vi "Unit Test - Copy Specified State.vi"() -> (3 "Array":T1(array[cluster])=[{"state"="Idle", "error out"={"status"=FALSE, "code"=0, "source"=""}, "Execution:State"=enum."Idle"}, {"state"="CSM Documentation", "error out"={"status"=FALSE, "code"=0, "source"=""}, "Execution:State"=enum."Idle"}, {"state"="VI Reference", "error out"={"status"=FALSE, "code"=0, "source"=""}, "Execution:State"=enum."Idle"}, {"state"="Error Handler", "error out"={"status"=FALSE, "code"=0, "source"=""}, "Execution:State"=enum."Bad"}, {"state"="Critical Error", "error out"={"status"=FALSE, "code"=0, "source"=""}, "Execution:State"=enum."Idle"}, {"state"="Target Timeout Error", "error out"={"status"=FALSE, "code"=0, "source"=""}, "Execution:State"=enum."Idle"}, {"state"="Target Error", "error out"={"status"=FALSE, "code"=0, "source"=""}, "Execution:State"=enum."Idle"}, {"state"="Async Response", "error out"={"status"=FALSE, "code"=0, "source"=""}, "Execution:State"=enum."Idle"}, {"state"="Response", "error out"={"status"=FALSE, "code"=0, "source"=""}, "Execution:State"=enum."Idle"}, {"state"="Async Message Posted", "error out"={"status"=FALSE, "code"=0, "source"=""}, "Execution:State"=enum."Idle"}, {"state"="Initialize Core Data", "error out"={"status"=FALSE, "code"=0, "source"=""}, "Execution:State"=enum."Idle"}, {"state"="Exit", "error out"={"status"=FALSE, "code"=0, "source"=""}, "Execution:State"=enum."Idle"}, {"state"="Data: Initialize", "error out"={"status"=FALSE, "code"=0, "source"=""}, "Execution:State"=enum."Idle"}, {"state"="Data: Update Indicators", "error out"={"status"=FALSE, "code"=0, "source"=""}, "Execution:State"=enum."Idle"}, {"state"="Data: Cleanup", "error out"={"status"=FALSE, "code"=0, "source"=""}, "Execution:State"=enum."Idle"}, {"state"="Macro: Initialize", "error out"={"status"=FALSE, "code"=0, "source"=""}, "Execution:State"=enum."Idle"}, {"state"="Macro: Exit", "error out"={"status"=FALSE, "code"=0, "source"=""}, "Execution:State"=enum."Idle"}, {"state"="API: API1", "error out"={"status"=FALSE, "code"=0, "source"=""}, "Execution:State"=enum."Idle"}, {"state"="API: API2", "error out"={"status"=FALSE, "code"=0, "source"=""}, "Execution:State"=enum."Idle"}, {"state"="Action: action1", "error out"={"status"=FALSE, "code"=0, "source"=""}, "Execution:State"=enum."Idle"}, {"state"="Action: action2", "error out"={"status"=FALSE, "code"=0, "source"=""}, "Execution:State"=enum."Idle"}])   [LabVIEW 2017, in "testcase-csmhelper.lvclass"]
uses:
  testcase-csmhelper.lvclass
  src/user.lib/_NEVSTOP/Communicable State Machine(CSM)/_csmHelper/CSM-Helper.lvclass/CSM-Helper.ctl
  src/user.lib/_NEVSTOP/Communicable State Machine(CSM)/_csmHelper/Properties/Read VI Ref.vi
  src/user.lib/_NEVSTOP/Communicable State Machine(CSM)/_csmHelper/API/Create From VI Reference.vi
  src/user.lib/_NEVSTOP/Communicable State Machine(CSM)/_csmHelper/API/Start Undo.vi
  src/user.lib/_NEVSTOP/Communicable State Machine(CSM)/_csmHelper/API/Copy State.vi
  src/user.lib/_NEVSTOP/Communicable State Machine(CSM)/_csmHelper/API/Stop Undo.vi
  src/user.lib/_NEVSTOP/Communicable State Machine(CSM)/_csmHelper/API/Undo.vi
  src/user.lib/_NEVSTOP/Communicable State Machine(CSM)/_csmHelper/API/Destroy.vi
  src/user.lib/_NEVSTOP/Communicable State Machine(CSM)/_csmHelper/CSM-Helper.lvclass
  src/user.lib/_NEVSTOP/Communicable State Machine(CSM)/_csmHelper/API/Open Block Diagram.vi
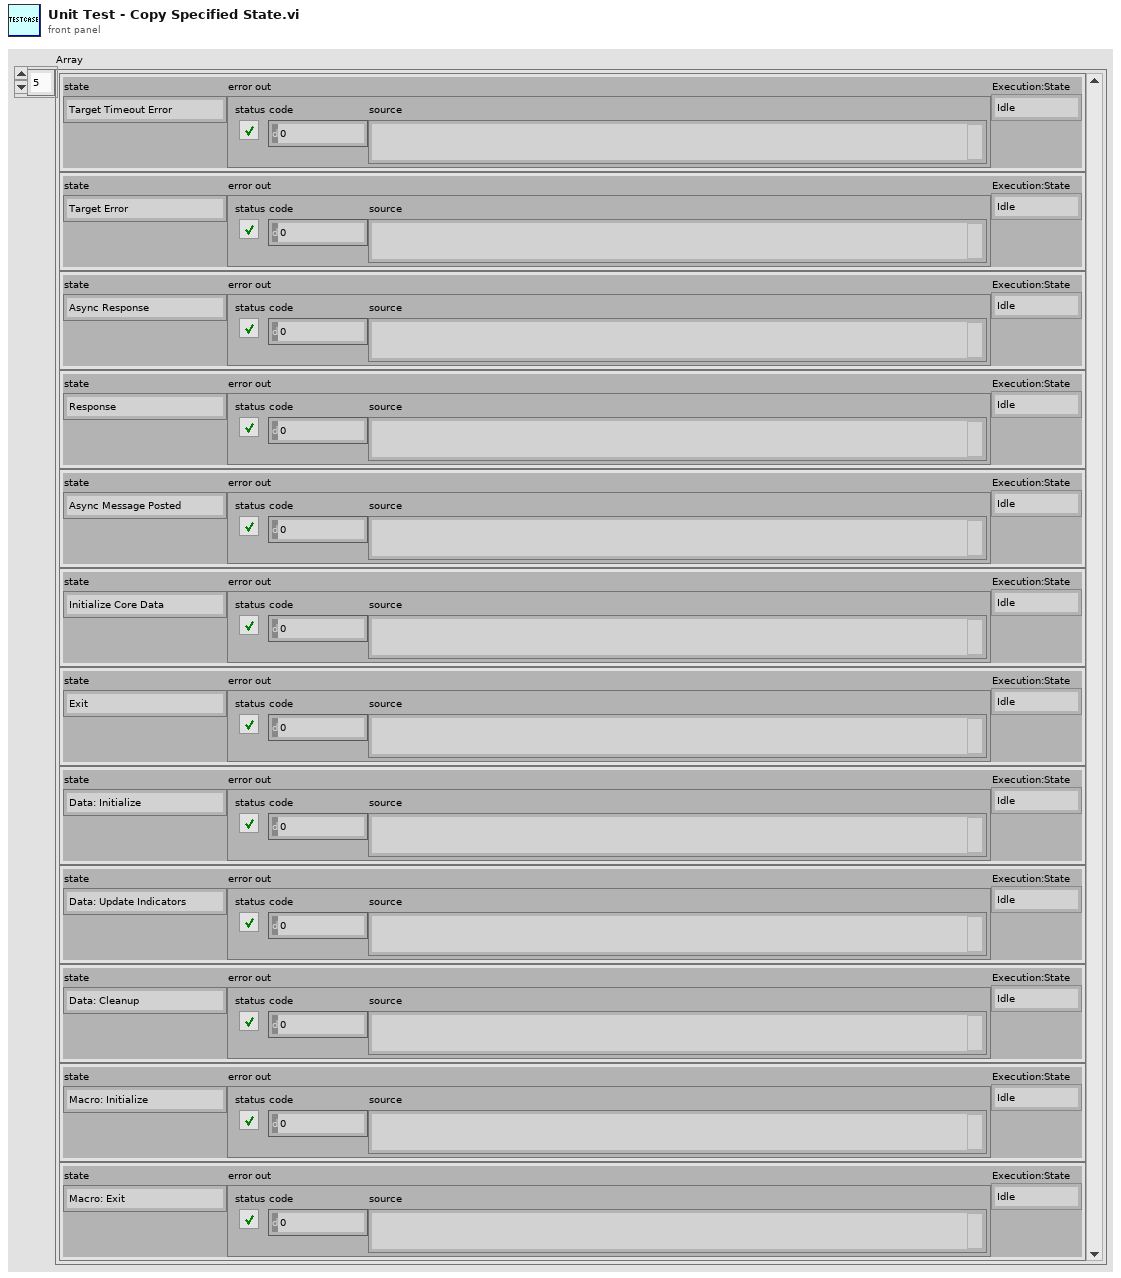
[diagram p1: front panel]
types:
  T1 = cluster{"state":string, "error out":errorcluster, "Execution:State":enum32{"Bad", "Idle", "Run top level", "Running"}}[]
  T2 = enum32{"Bad", "Idle", "Run top level", "Running"}
  T3 = cluster{string, "error out":errorcluster, "Exec.State":enum32{"Bad", "Idle", "Run top level", "Running"}}
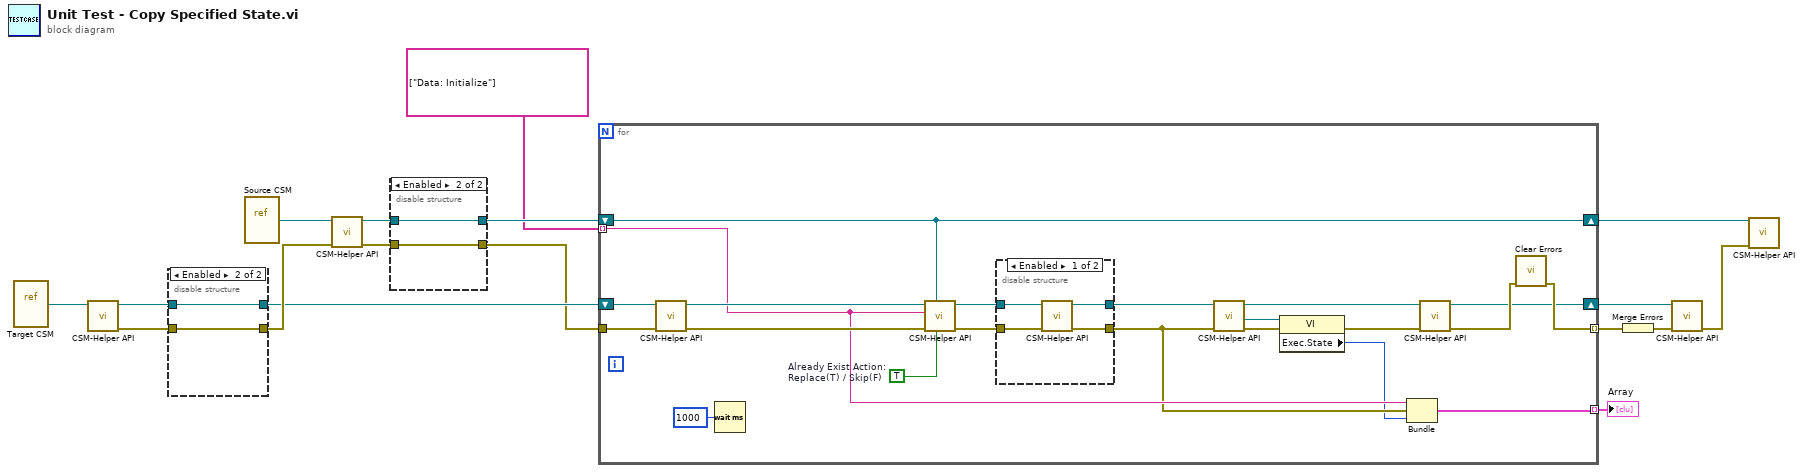
[diagram p0: block diagram]
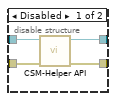
[diagram p2: hidden frame]
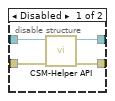
[diagram p3: hidden frame]
diagram:
  n1 = vi-ref "Target CSM.vi"() -> (w1:refnum<vi>)
  n2 = call-poly "CSM-Helper API.vi"("VI"=w1) -> ("error out"=w15:errorcluster, "CSM-Helper.lvclass"=w14:refnum<class "CSM-Helper.lvclass">)  [unwired: 9 in]
  n3 = disable-structure shown="Enabled" {
    disable-tunnel: w15 -> [w21 w22]
    disable-tunnel: w14 -> [w20 w23]
    disable-tunnel: [w19 w22] -> w11
    disable-tunnel: [w18 w23] -> w10
    frame Disabled {
      n4 = call-poly "CSM-Helper API.vi"("error in (no error)"=w21, "CSM-Helper in"=w20) -> ("error out"=w19:errorcluster, "CSM-Helper out"=w18:refnum<class "CSM-Helper.lvclass">)  [unwired: 8 in]
    }
    frame Enabled {
    }
  }
  n5 = vi-ref "Source CSM.vi"() -> (w2:refnum<vi>)
  n6 = call-poly "CSM-Helper API.vi"("error in (no error)"=w11, "VI"=w2) -> ("error out"=w12:errorcluster, "CSM-Helper.lvclass"=w13:refnum<class "CSM-Helper.lvclass">)  [unwired: 8 in]
  n7 = disable-structure shown="Enabled" {
    disable-tunnel: w13 -> [w27 w29]
    disable-tunnel: w12 -> [w26 w28]
    disable-tunnel: [w25 w29] -> w5
    disable-tunnel: [w24 w28] -> w4
    frame Disabled {
      n8 = call-poly "CSM-Helper API.vi"("error in (no error)"=w26, "CSM-Helper in"=w27) -> ("error out"=w24:errorcluster, "CSM-Helper out"=w25:refnum<class "CSM-Helper.lvclass">)  [unwired: 8 in]
    }
    frame Enabled {
    }
  }
  n9 = for {
    shift-right: [w38] -> w17
    shift-left: w10 -> [w49]
    shift-right: [w44] -> w8
    shift-left: w5 -> [w44]
    tunnel: string[] ["Data: Initialize"] ("Value") -> [w42] mode=indexing
    tunnel: w4 -> [w48]
    tunnel: [w43] -> w16 mode=indexing
    tunnel: [w41] -> w6 mode=indexing
    w30 = TRUE  # Already Exist Action: Replace(T) / Skip(F)
    n10 = call-poly "CSM-Helper API.vi"("error in (no error)"=w48, "CSM-Helper in"=w49) -> ("error out"=w47:errorcluster, "CSM-Helper out"=w46:refnum<class "CSM-Helper.lvclass">)  [unwired: 8 in]
    n11 = Wait (ms)(milliseconds to wait=u32 1000) -> ()  [unwired: 1 out]
    n12 = call-poly "CSM-Helper API.vi"("Already Exist Action:\nReplace(T) / Skip(F)"=w30, "SourceCSM"=w44, "error in (no error)"=w47, "Case"=w42, "CSM-Helper.lvclass"=w46) -> ("error out"=w45:errorcluster, "CSM-Helper out 2"=w50:refnum<class "CSM-Helper.lvclass">)  [unwired: 5 in]
    n13 = disable-structure shown="Enabled" {
      disable-tunnel: [w54 w56] -> w36
      disable-tunnel: w45 -> [w53 w55]
      disable-tunnel: [w52 w55] -> w37
      disable-tunnel: w50 -> [w51 w56]
      frame Enabled {
        n14 = call-poly "CSM-Helper API.vi"("error in (no error)"=w53, "CSM-Helper in"=w51) -> ("error out"=w52:errorcluster, "CSM-Helper out"=w54:refnum<class "CSM-Helper.lvclass">)  [unwired: 8 in]
      }
      frame Disabled {
      }
    }
    n15 = call-poly "CSM-Helper API.vi"("error in (no error)"=w37, "CSM-Helper in"=w36) -> ("error out"=w34:errorcluster, "VI"=w32:refnum<vi>, "CSM-Helper out"=w35:refnum<class "CSM-Helper.lvclass">)  [unwired: 7 in]
    n16 = property class="VI"(reference=w32, error in=w34) -> (error out=w33:errorcluster, "Exec.State"=w31:T2)  [unwired: 1 out]
    n17 = Bundle(w42, "error out"=w37, "Exec.State"=w31) -> (w41:T3)  [unwired: 1 in]
    n18 = call-poly "CSM-Helper API.vi"("error in (no error)"=w33, "CSM-Helper in"=w35) -> ("error out"=w39:errorcluster, "CSM-Helper out"=w38:refnum<class "CSM-Helper.lvclass">)  [unwired: 8 in]
    n19 = call <vilib>:"Clear Errors.vi"("error in (no error)"=w39) -> ("error out"=w43:errorcluster)  [unwired: 5 in, 1 out]
  }
  "Array" <- w6
  n20 = Merge Errors(w16) -> (w7:errorcluster)
  n21 = call-poly "CSM-Helper API.vi"("error in (no error)"=w7, "CSM-Helper in"=w17) -> ("error out"=w9:errorcluster)  [unwired: 8 in, 1 out]
  n22 = call-poly "CSM-Helper API.vi"("error in (no error)"=w9, "CSM-Helper in"=w8) -> ()  [unwired: 8 in, 2 out]
